vi "TCS_emul.vi"() -> ()   [LabVIEW 2011]
uses:
  <vilib>/Instr/_visa.llb/VISA Configure Serial Port (Instr).vi
panel:
  in  "ShowTraffic":bool
  out "error out":errorcluster
  out "error out":errorcluster
  in  "TCS R Baud":u32=57600
  in  "TCS R VRN":refnum<visa-resource-name>="COM10"
  in  "STATEX":bool[](array[boolean])=[FALSE, FALSE, FALSE, FALSE, FALSE, FALSE, FALSE, FALSE]
  in  "STATLH":bool[](array[boolean])=[FALSE, FALSE, FALSE, FALSE, FALSE, FALSE, FALSE, FALSE]
  in  "STATH":bool[](array[boolean])=[FALSE, FALSE, FALSE, FALSE, FALSE, FALSE, FALSE, TRUE]
  in  "STATL":bool[](array[boolean])=[TRUE, FALSE, TRUE, FALSE, TRUE, FALSE, FALSE, FALSE]
  in  "Rotator":dbl=90.0 format="%.2f"
  in  "Dome":dbl=140.0 format="%.2f"
  in  "Focus":dbl=3200.0 format="%.2f"
  out "All Tx":string
  out "All Rx":string
  in  "QUIT":bool
  in  "TCS C Baud":u32=57600
  in  "TCS C Baud":refnum<visa-resource-name>="COM6"
  in  "Air Mass":dbl=2.122384 format="%.3f"
  in  "RA Tel":dbl caption="Asc. Droite" format="%<%H:%M:%S%1u>t"
  in  "DEC Tel":dbl=36000.0 caption="Déclinaison" format="%<%H:%M:%S%0u>t"
  in  "Angle Hor.":dbl format="%<%H:%M:%S%0u>t"
  in  "Epoch Tel":dbl=2000.0 caption="Époque" format="%.2f"
  out "UTC":dbl=67576.0 caption="Temps Univ." format="%<%H:%M:%S%0u>t"
  out "LST":dbl=8878.983717685333 caption="Temps Sidé." format="%<%H:%M:%S%0u>t"
  # "Télescope"
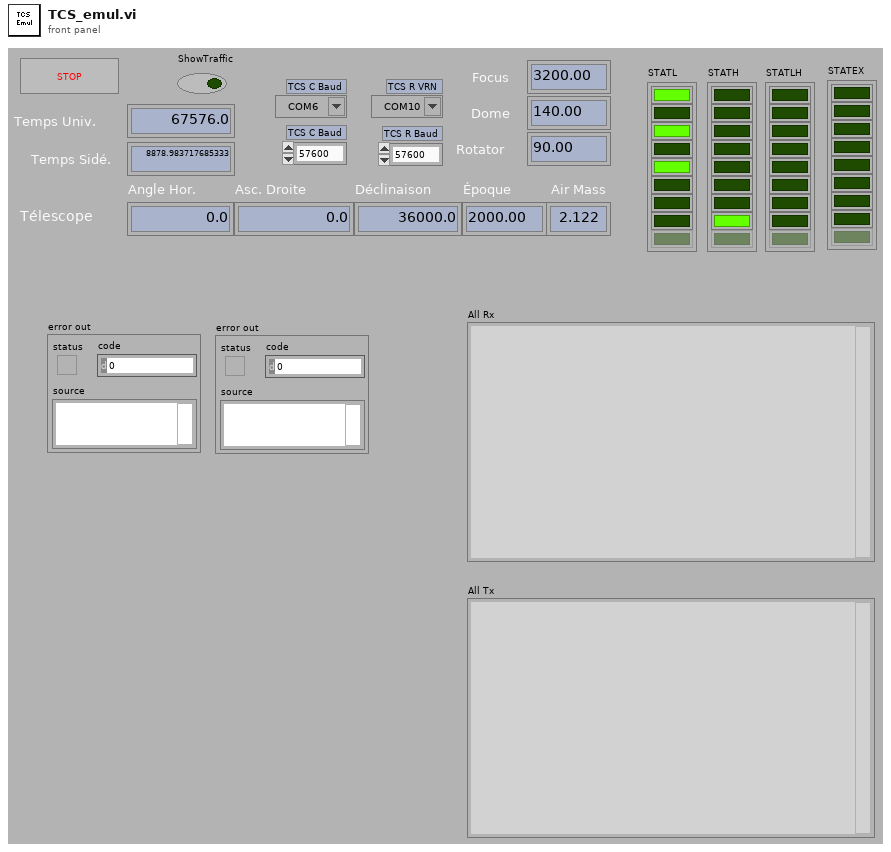
[diagram p1: front panel]
types:
  T1 = typedef "LVDateTimeRec.ctl" = cluster{"fractional second":dbl, "second":i32, "minute":i32, "hour":i32, "day of month":i32, "month":i32, "year":i32, "day of week":i32, "day of year":i32, "DST":i32}
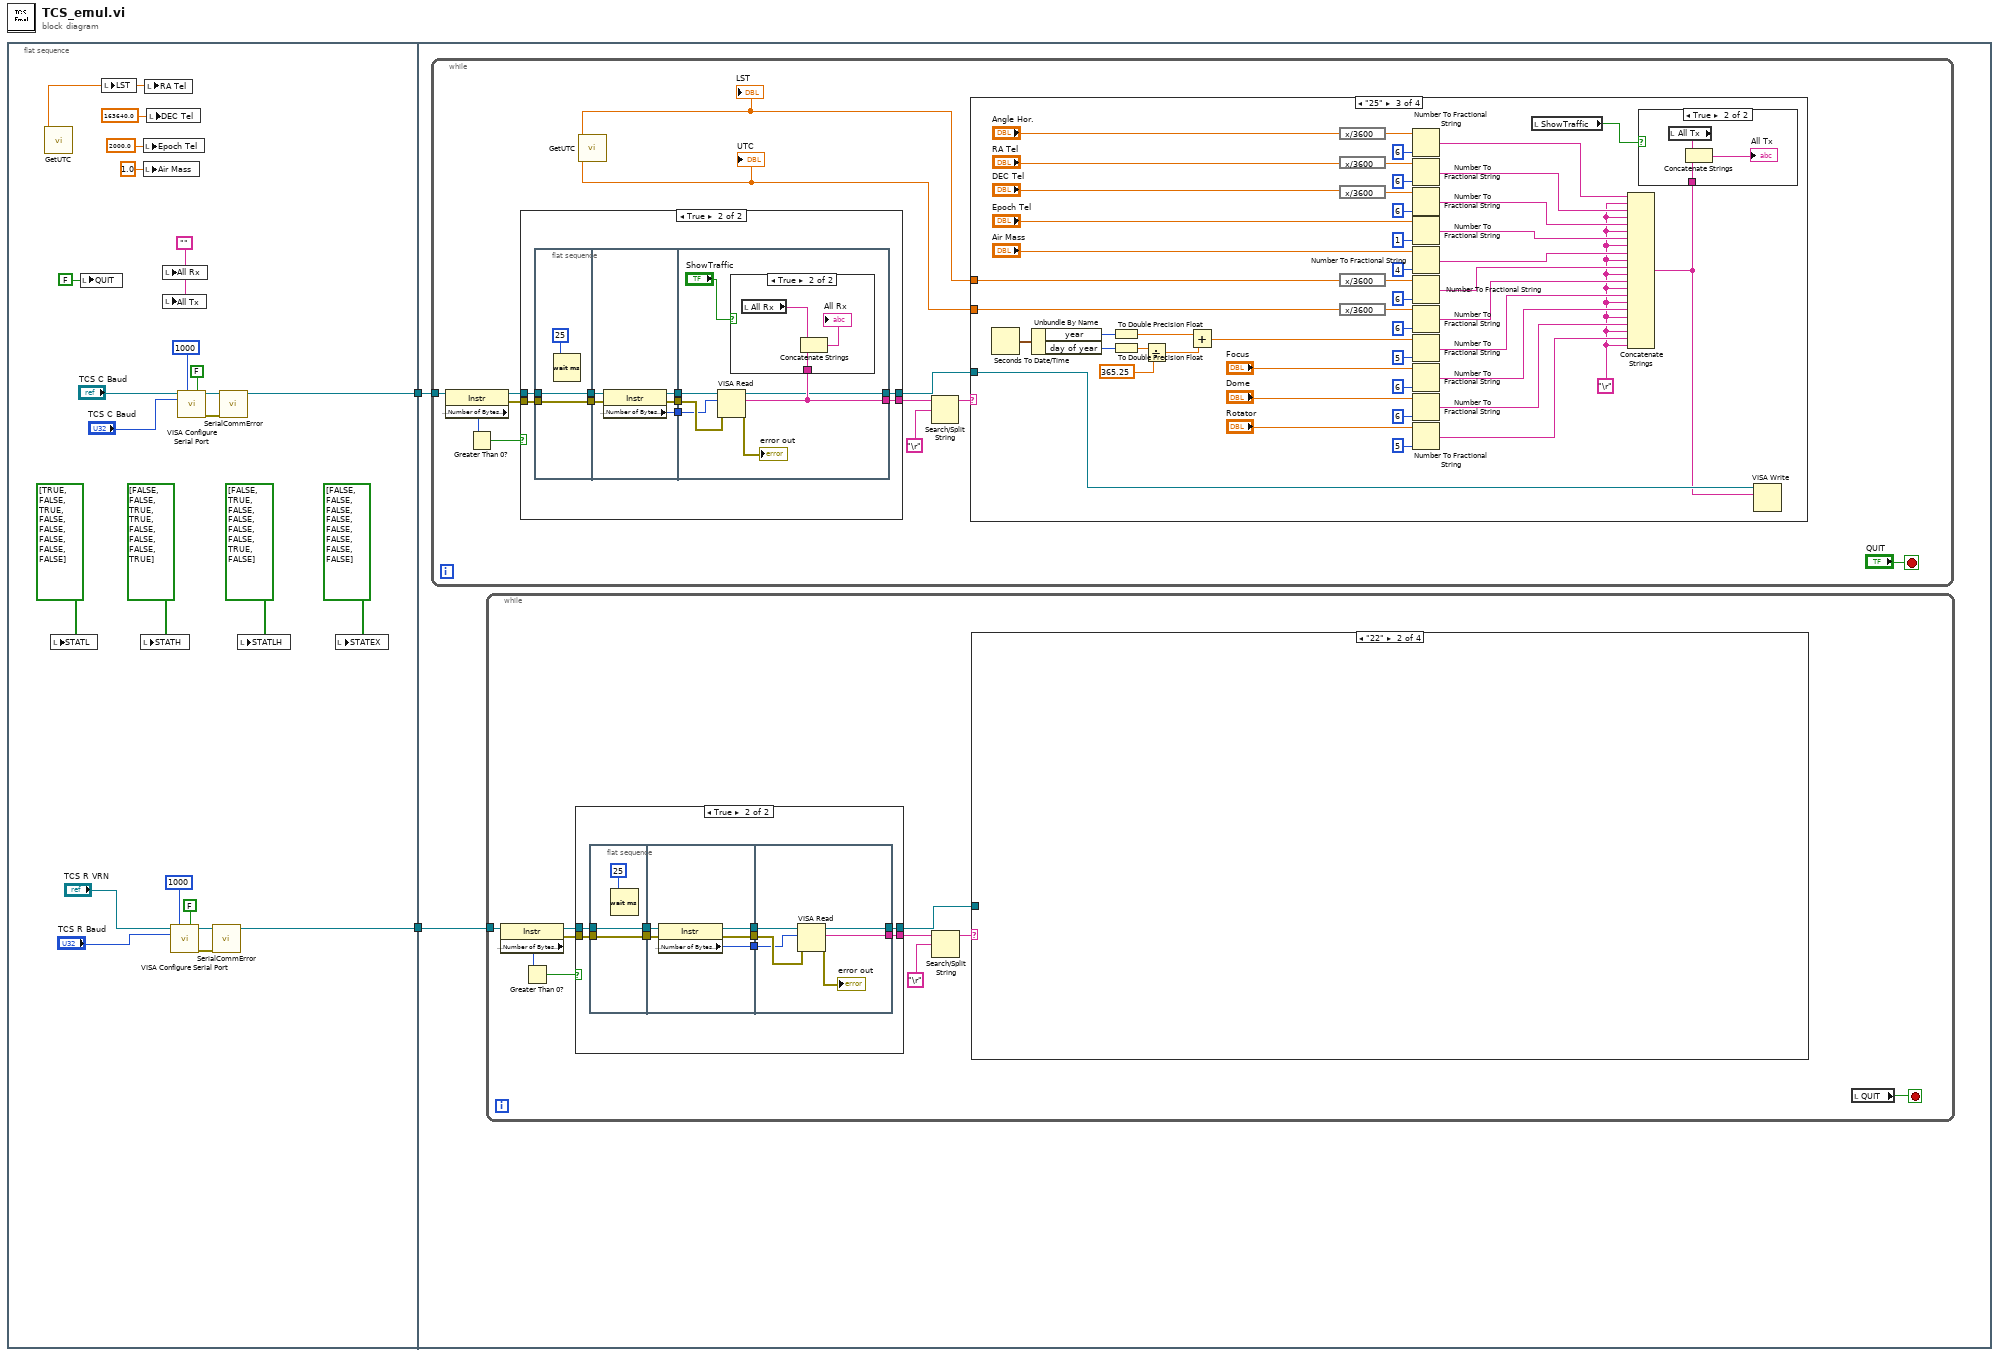
[diagram p0: block diagram]
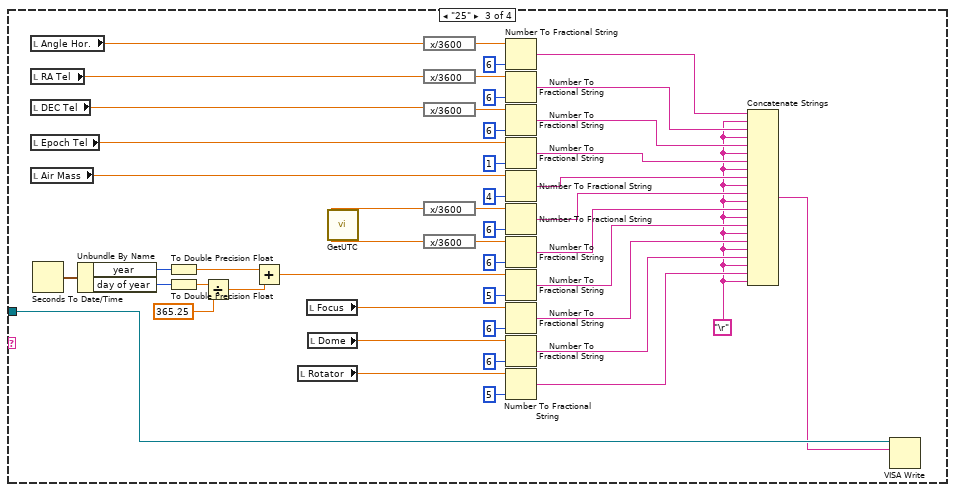
[diagram p3: hidden frame]
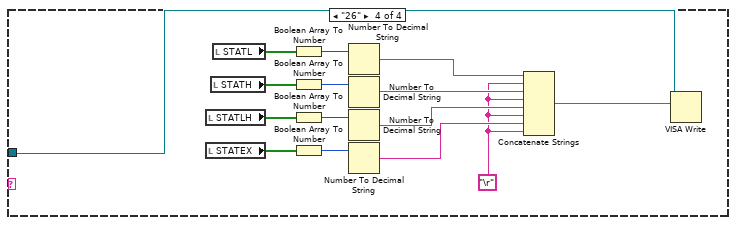
[diagram p4: hidden frame]
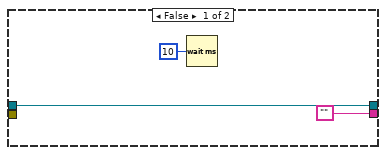
[diagram p5: hidden frame]
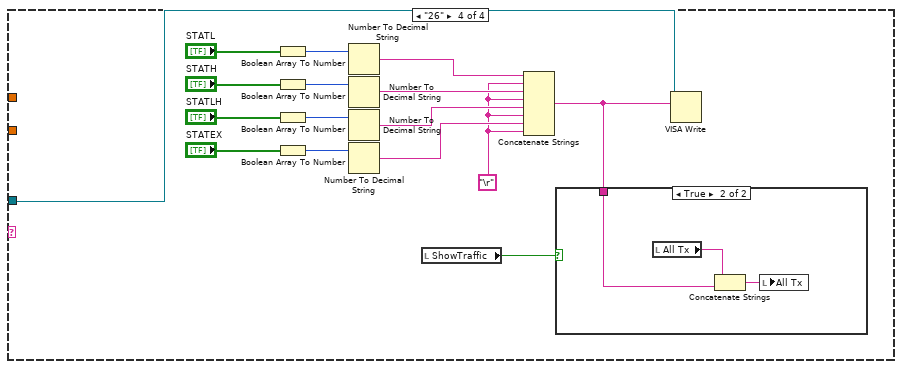
[diagram p9: hidden frame]
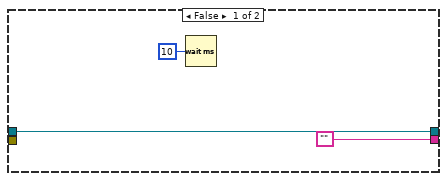
[diagram p11: hidden frame]
diagram:
  n1 = flat-sequence {
    tunnel: [w8] -> w2
    tunnel: [w7] -> w1
    tunnel: w2 -> [w28]
    tunnel: w1 -> [w27]
    frame #0 {
      w20 = ""
      n2 = call "GetUTC.vi"() -> ("LST+_seconds"=w6:dbl)  [unwired: 7 out]
      n3 = local write "STATL"(bool[] [TRUE, FALSE, TRUE, FALSE, FALSE, FALSE, FALSE, FALSE] ("STATEX")) -> ()
      n4 = local write "QUIT"(FALSE ("QUIT")) -> ()
      n5 = local write "LST"(w6) -> ()
      n6 = local write "STATH"(bool[] [FALSE, FALSE, TRUE, TRUE, FALSE, FALSE, FALSE, TRUE] ("STATEX")) -> ()
      n7 = local write "Epoch Tel"(2000.0 ("Epoch Tel")) -> ()
      n8 = local write "Air Mass"(1.0 ("Air Mass")) -> ()
      n9 = local write "RA Tel"(w6) -> ()
      n10 = local write "DEC Tel"(163640.0 ("DEC Tel")) -> ()
      n11 = local write "All Rx"(w20) -> ()
      n12 = local write "All Tx"(w20) -> ()
      n13 = call-poly "VISA Configure Serial Port"("VISA resource name"="TCS R VRN", "timeout (10sec)"=u32 1000, "Enable Termination\nChar (T)"=FALSE ("Enable Termination\nChar (T)"), "baud rate (9600)"="TCS R Baud") -> ("VISA resource name out"=w18:refnum<visa-resource-name>, "error out"=w19:errorcluster)  [unwired: 10 in]
      n14 = call-poly "VISA Configure Serial Port"("VISA resource name"="TCS C Baud", "timeout (10sec)"=u32 1000, "Enable Termination\nChar (T)"=FALSE ("Enable Termination\nChar (T)"), "baud rate (9600)"="TCS C Baud") -> ("VISA resource name out"=w24:refnum<visa-resource-name>, "error out"=w23:errorcluster)  [unwired: 10 in]
      n15 = call "SerialCommError.vi"("VISA IN"=w18, "error IN"=w19) -> ("VISA OUT"=w7:refnum<visa-resource-name>)  [unwired: 11 in, 2 out]
      n16 = call "SerialCommError.vi"("VISA IN"=w24, "error IN"=w23) -> ("VISA OUT"=w8:refnum<visa-resource-name>)  [unwired: 11 in, 2 out]
      n17 = local write "STATLH"(bool[] [FALSE, TRUE, FALSE, FALSE, FALSE, FALSE, TRUE, FALSE] ("STATEX")) -> ()
      n18 = local write "STATEX"(bool[] [FALSE, FALSE, FALSE, FALSE, FALSE, FALSE, FALSE, FALSE] ("STATEX")) -> ()
    }
    frame #1 {
      n19 = while {
        tunnel: w28 -> [w139]
        stop <- "QUIT" stop-if-true
        n20 = property class="Instr"(reference=w139) -> (reference out=w136:refnum<visa-resource-name>, error out=w135:errorcluster, "Serial Settings:Number of Bytes at Serial Port"=w137:u32)  [unwired: 1 in]
        n21 = Greater Than 0?(x=w137) -> (x > 0?=w138:bool)
        n22 = case shown="True" w138 {
          tunnel: w136 -> [w212 w222]
          tunnel: w135 -> [_ w221]
          tunnel: ["" w219] -> w133
          tunnel: [w212 w218] -> w130
          frame False {
            n23 = Wait (ms)(milliseconds to wait=u32 10) -> ()  [unwired: 1 out]
          }
          frame True {
            n24 = flat-sequence {
              tunnel: w221 -> [w224]
              tunnel: w222 -> [w225]
              tunnel: [w225] -> w215
              tunnel: [w224] -> w214
              tunnel: [w228] -> w220
              tunnel: [w227] -> w217
              tunnel: [w226] -> w216
              tunnel: w215 -> [w230]
              tunnel: w214 -> [w229]
              tunnel: w220 -> [w237]
              tunnel: [w235] -> w219
              tunnel: [w234] -> w218
              tunnel: w217 -> [w236]
              tunnel: w216 -> [w233]
              frame #0 {
                n25 = Wait (ms)(milliseconds to wait=u32 25) -> ()  [unwired: 1 out]
              }
              frame #1 {
                n26 = property class="Instr"(reference=w230, error in=w229) -> (reference out=w228:refnum<visa-resource-name>, error out=w227:errorcluster, "Serial Settings:Number of Bytes at Serial Port"=w226:u32)
              }
              frame #2 {
                n27 = VISA Read(VISA resource name=w237, byte count=w233, error in (no error)=w236) -> (VISA resource name out=w234:refnum<visa-resource-name>, read buffer=w235:string, error out=→"error out":errorcluster)  [unwired: 1 out]
                n28 = case shown="True" "ShowTraffic" {
                  tunnel: w235 -> [_ w239]
                  frame False {
                  }
                  frame True {
                    n29 = local read "All Rx"() -> (w240:string)
                    n30 = Concatenate Strings(w240, w239) -> (→"All Rx":string)
                  }
                }
              }
            }
          }
        }
        n31 = call "GetUTC.vi"() -> ("LST+_seconds"=w129:dbl, "UTC_seconds"=w128:dbl)  [unwired: 6 out]
        "LST" <- w129
        "UTC" <- w128
        n32 = Search/Split String(string=w133, search string/char (-)="\r") -> (substring before match=w131:string)  [unwired: 1 in, 2 out]
        n33 = case shown="\"25\"" w131 {
          tunnel: w130 -> [_ _ w144 w194]
          tunnel: w129 -> [_ _ w142 _]
          tunnel: w128 -> [_ _ w141 _]
          frame "", Default {
          }
          frame "22" {
          }
          frame "25" {
            w145 = "\r"
            n34 = Seconds To Date/Time() -> (date time rec=w188:T1)  [unwired: 2 in]
            n35 = Unbundle By Name(w188) -> ("year"=w185:i32, "day of year"=w187:i32)
            n36 = To Double Precision Float(number=w185) -> (double precision float=w183:dbl)
            n37 = To Double Precision Float(number=w187) -> (double precision float=w186:dbl)
            n38 = Divide(x=w186, y=365.25) -> (x/y=w182:dbl)
            n39 = Add(x=w183, y=w182) -> (x+y=w157:dbl)
            n40 = expression code="x/3600"("Angle Hor.") -> (w181:dbl)
            n41 = expression code="x/3600"("RA Tel") -> (w179:dbl)
            n42 = expression code="x/3600"("DEC Tel") -> (w177:dbl)
            n43 = expression code="x/3600"(w142) -> (w167:dbl)
            n44 = expression code="x/3600"(w141) -> (w165:dbl)
            n45 = Number To Fractional String(number=w181, precision (6)=i16 6 ("width (-)")) -> (F-format string=w156:string)  [unwired: 2 in]
            n46 = Number To Fractional String(number=w179, precision (6)=i16 6 ("width (-)")) -> (F-format string=w155:string)  [unwired: 2 in]
            n47 = Number To Fractional String(number=w177, precision (6)=i16 6 ("width (-)")) -> (F-format string=w154:string)  [unwired: 2 in]
            n48 = Number To Fractional String(number="Epoch Tel", precision (6)=i16 1 ("width (-)")) -> (F-format string=w153:string)  [unwired: 2 in]
            n49 = Number To Fractional String(number="Air Mass", precision (6)=i16 4 ("width (-)")) -> (F-format string=w152:string)  [unwired: 2 in]
            n50 = Number To Fractional String(number=w167, precision (6)=i16 6 ("width (-)")) -> (F-format string=w151:string)  [unwired: 2 in]
            n51 = Number To Fractional String(number=w165, precision (6)=i16 6 ("width (-)")) -> (F-format string=w150:string)  [unwired: 2 in]
            n52 = Number To Fractional String(number=w157, precision (6)=i16 5 ("width (-)")) -> (F-format string=w149:string)  [unwired: 2 in]
            n53 = Number To Fractional String(number="Focus", precision (6)=i16 6 ("width (-)")) -> (F-format string=w148:string)  [unwired: 2 in]
            n54 = Number To Fractional String(number="Dome", precision (6)=i16 6 ("width (-)")) -> (F-format string=w147:string)  [unwired: 2 in]
            n55 = Number To Fractional String(number="Rotator", precision (6)=i16 5 ("width (-)")) -> (F-format string=w146:string)  [unwired: 2 in]
            n56 = local read "ShowTraffic"() -> (w140:bool)
            n57 = Concatenate Strings(w156, w145, w155, w145, w154, w145, w153, w145, w152, w145, w151, w145, w150, w145, w149, w145, w148, w145, w147, w145, w146, w145) -> (w143:string)
            n58 = case shown="True" w140 {
              tunnel: w143 -> [_ w189]
              frame False {
              }
              frame True {
                n59 = local read "All Tx"() -> (w191:string)
                n60 = Concatenate Strings(w191, w189) -> (→"All Tx":string)
              }
            }
            n61 = VISA Write(VISA resource name=w144, write buffer=w143) -> ()  [unwired: 1 in, 3 out]
          }
          frame "26" {
            w195 = "\r"
            n62 = Boolean Array To Number(Boolean array="STATL") -> (number=w207:u32)
            n63 = Boolean Array To Number(Boolean array="STATH") -> (number=w205:u32)
            n64 = Boolean Array To Number(Boolean array="STATLH") -> (number=w204:u32)
            n65 = Boolean Array To Number(Boolean array="STATEX") -> (number=w203:u32)
            n66 = Number To Decimal String(number=w207) -> (decimal integer string=w199:string)  [unwired: 1 in]
            n67 = Number To Decimal String(number=w205) -> (decimal integer string=w198:string)  [unwired: 1 in]
            n68 = Number To Decimal String(number=w204) -> (decimal integer string=w197:string)  [unwired: 1 in]
            n69 = Number To Decimal String(number=w203) -> (decimal integer string=w196:string)  [unwired: 1 in]
            n70 = local read "ShowTraffic"() -> (w192:bool)
            n71 = Concatenate Strings(w199, w195, w198, w195, w197, w195, w196, w195) -> (w193:string)
            n72 = case shown="True" w192 {
              tunnel: w193 -> [_ w208]
              frame False {
              }
              frame True {
                n73 = local read "All Tx"() -> (w209:string)
                n74 = Concatenate Strings(w209, w208) -> (w210:string)
                n75 = local write "All Tx"(w210) -> ()
              }
            }
            n76 = VISA Write(VISA resource name=w194, write buffer=w193) -> ()  [unwired: 1 in, 3 out]
          }
        }
      }
      n77 = while {
        tunnel: w27 -> [w38]
        stop <- w29 stop-if-true
        n78 = property class="Instr"(reference=w38) -> (reference out=w35:refnum<visa-resource-name>, error out=w34:errorcluster, "Serial Settings:Number of Bytes at Serial Port"=w36:u32)  [unwired: 1 in]
        n79 = Greater Than 0?(x=w36) -> (x > 0?=w37:bool)
        n80 = case shown="True" w37 {
          tunnel: w35 -> [w103 w113]
          tunnel: w34 -> [_ w112]
          tunnel: ["" w110] -> w33
          tunnel: [w103 w109] -> w30
          frame False {
            n81 = Wait (ms)(milliseconds to wait=u32 10) -> ()  [unwired: 1 out]
          }
          frame True {
            n82 = flat-sequence {
              tunnel: w112 -> [w115]
              tunnel: w113 -> [w116]
              tunnel: [w116] -> w106
              tunnel: [w115] -> w105
              tunnel: [w119] -> w111
              tunnel: [w118] -> w108
              tunnel: [w117] -> w107
              tunnel: w106 -> [w121]
              tunnel: w105 -> [w120]
              tunnel: w111 -> [w127]
              tunnel: [w125] -> w110
              tunnel: [w124] -> w109
              tunnel: w108 -> [w126]
              tunnel: w107 -> [w123]
              frame #0 {
                n83 = Wait (ms)(milliseconds to wait=u32 25) -> ()  [unwired: 1 out]
              }
              frame #1 {
                n84 = property class="Instr"(reference=w121, error in=w120) -> (reference out=w119:refnum<visa-resource-name>, error out=w118:errorcluster, "Serial Settings:Number of Bytes at Serial Port"=w117:u32)
              }
              frame #2 {
                n85 = VISA Read(VISA resource name=w127, byte count=w123, error in (no error)=w126) -> (VISA resource name out=w124:refnum<visa-resource-name>, read buffer=w125:string, error out=→"error out":errorcluster)  [unwired: 1 out]
              }
            }
          }
        }
        n86 = Search/Split String(string=w33, search string/char (-)="\r") -> (substring before match=w31:string)  [unwired: 1 in, 2 out]
        n87 = case shown="\"22\"" w31 {
          tunnel: w30 -> [_ _ w50 w92]
          frame "", Default {
          }
          frame "22" {
          }
          frame "25" {
            w51 = "\r"
            n88 = local read "Angle Hor."() -> (w48:dbl)
            n89 = local read "RA Tel"() -> (w41:dbl)
            n90 = local read "DEC Tel"() -> (w42:dbl)
            n91 = local read "Epoch Tel"() -> (w43:dbl)
            n92 = local read "Air Mass"() -> (w44:dbl)
            n93 = Seconds To Date/Time() -> (date time rec=w86:T1)  [unwired: 2 in]
            n94 = Unbundle By Name(w86) -> ("year"=w83:i32, "day of year"=w85:i32)
            n95 = To Double Precision Float(number=w83) -> (double precision float=w81:dbl)
            n96 = To Double Precision Float(number=w85) -> (double precision float=w84:dbl)
            n97 = Divide(x=w84, y=365.25) -> (x/y=w80:dbl)
            n98 = Add(x=w81, y=w80) -> (x+y=w63:dbl)
            n99 = local read "Rotator"() -> (w45:dbl)
            n100 = local read "Focus"() -> (w47:dbl)
            n101 = local read "Dome"() -> (w46:dbl)
            n102 = call "GetUTC.vi"() -> ("LST+_seconds"=w40:dbl, "UTC_seconds"=w39:dbl)  [unwired: 6 out]
            n103 = expression code="x/3600"(w48) -> (w79:dbl)
            n104 = expression code="x/3600"(w41) -> (w78:dbl)
            n105 = expression code="x/3600"(w42) -> (w77:dbl)
            n106 = expression code="x/3600"(w40) -> (w70:dbl)
            n107 = expression code="x/3600"(w39) -> (w68:dbl)
            n108 = Number To Fractional String(number=w79, precision (6)=i16 6 ("width (-)")) -> (F-format string=w62:string)  [unwired: 2 in]
            n109 = Number To Fractional String(number=w78, precision (6)=i16 6 ("width (-)")) -> (F-format string=w61:string)  [unwired: 2 in]
            n110 = Number To Fractional String(number=w77, precision (6)=i16 6 ("width (-)")) -> (F-format string=w60:string)  [unwired: 2 in]
            n111 = Number To Fractional String(number=w43, precision (6)=i16 1 ("width (-)")) -> (F-format string=w59:string)  [unwired: 2 in]
            n112 = Number To Fractional String(number=w44, precision (6)=i16 4 ("width (-)")) -> (F-format string=w58:string)  [unwired: 2 in]
            n113 = Number To Fractional String(number=w70, precision (6)=i16 6 ("width (-)")) -> (F-format string=w57:string)  [unwired: 2 in]
            n114 = Number To Fractional String(number=w68, precision (6)=i16 6 ("width (-)")) -> (F-format string=w56:string)  [unwired: 2 in]
            n115 = Number To Fractional String(number=w63, precision (6)=i16 5 ("width (-)")) -> (F-format string=w55:string)  [unwired: 2 in]
            n116 = Number To Fractional String(number=w47, precision (6)=i16 6 ("width (-)")) -> (F-format string=w54:string)  [unwired: 2 in]
            n117 = Number To Fractional String(number=w46, precision (6)=i16 6 ("width (-)")) -> (F-format string=w53:string)  [unwired: 2 in]
            n118 = Number To Fractional String(number=w45, precision (6)=i16 5 ("width (-)")) -> (F-format string=w52:string)  [unwired: 2 in]
            n119 = Concatenate Strings(w62, w51, w61, w51, w60, w51, w59, w51, w58, w51, w57, w51, w56, w51, w55, w51, w54, w51, w53, w51, w52, w51) -> (w49:string)
            n120 = VISA Write(VISA resource name=w50, write buffer=w49) -> ()  [unwired: 1 in, 3 out]
          }
          frame "26" {
            w93 = "\r"
            n121 = local read "STATLH"() -> (w88:bool[])
            n122 = local read "STATEX"() -> (w87:bool[])
            n123 = local read "STATH"() -> (w89:bool[])
            n124 = local read "STATL"() -> (w90:bool[])
            n125 = Boolean Array To Number(Boolean array=w90) -> (number=w101:u32)
            n126 = Boolean Array To Number(Boolean array=w89) -> (number=w100:u32)
            n127 = Boolean Array To Number(Boolean array=w88) -> (number=w99:u32)
            n128 = Boolean Array To Number(Boolean array=w87) -> (number=w98:u32)
            n129 = Number To Decimal String(number=w101) -> (decimal integer string=w97:string)  [unwired: 1 in]
            n130 = Number To Decimal String(number=w100) -> (decimal integer string=w96:string)  [unwired: 1 in]
            n131 = Number To Decimal String(number=w99) -> (decimal integer string=w95:string)  [unwired: 1 in]
            n132 = Number To Decimal String(number=w98) -> (decimal integer string=w94:string)  [unwired: 1 in]
            n133 = Concatenate Strings(w97, w93, w96, w93, w95, w93, w94, w93) -> (w91:string)
            n134 = VISA Write(VISA resource name=w92, write buffer=w91) -> ()  [unwired: 1 in, 3 out]
          }
        }
        n135 = local read "QUIT"() -> (w29:bool)
      }
    }
  }
